vi "temp map test params.vi"() -> ()   [LabVIEW 2009]
uses:
  BME_DG_G05P2/SG05P2 Clock and Trigger Settings.ctl
  LV-BME Interface/BME_DG_TriggerSettings.ctl
  LV-BME Interface/ClockSource.ctl
  LV-BME Interface/BME_DG_V2TriggerSettings.ctl
  ChnlParam.ctl
  Chnl Settings Complete.ctl
  LV-BME Interface/ChnlSettings.ctl
  Go_Done_Chnl_Settings.ctl
  SG08_Chnl_Settings.ctl
  Card Config.ctl
  SG08_Settings.ctl
  POLARIS BME DG.lvlib
panel:
  in  "Advanced Chnl Settings":T1={"Go Signal"=16, "Done Signal"=16} {"Done Signal" format="%04x" items=["Local Primary"=1, "Local Secondary"=2, "Local Force"=4, "Master Primary"=16]; "Go Signal" format="%04x" items=["Local Primary"=1, "Local Secondary"=2, "Local Force"=4, "Resynchronize"=8, "Master Primary"=16, "Master Secondary"=32, "Master Force"=64, "System Clock"=128, "Delay Clock"=256, "Inhibit Local"=512, "Start Local"=1024, "Start Bus"=2048, "Step Back Local"=4096, "Step Back Bus"=8192, "From E"=65536, "From F"=131072, "From Bus"=262144]}
  in  "ChnParameter":T2={" Delay (µs)"=0.0, "On?"=TRUE, "PositiveVoltage?"=TRUE, "50OhmTerminated? "=TRUE, "25OhmOutput?"=FALSE} {"Delay (µs)" min=0.0 max=100000000.0 format="%.5f"}
  out "Card Config":T3[](array[typedef]) {"Advanced Settings"."Trigger on MS Bus" format="%04x" items=["Local Primary"=1, "Local Secondary"=2, "Local Force"=4, "Resynchronize"=8, "Master Primary"=16, "Master Secondary"=32, "Master Force"=64, "System Clock"=128, "Delay Clock"=256, "Inhibit Local"=512, "Start Local"=1024, "Start Bus"=2048, "Step Back Local"=4096, "Step Back Bus"=8192, "Enable From E"=65536, "Enable From F"=131072, "Enable From Bus"=262144]; "Advanced Settings"."Force Trigger (µs)" min=0.0 format="%.6f"; "SG08_Settings"."StepBackTime (µs)" min=0.0 format="%.6f"; "SG08_Settings"."Gate Delay (µs)" format="%.3f"; "SG08_Settings"."Gate Level" min=-2.5 max=2.5 format="%.3g"; "Base Settings"."Gate Divider" min=1 max=1000000; "Base Settings"."Clock Source" items=["Internal Oscillator"=1, "External Trigger"=2, "Trigger-> Oscillator"=3, "MasterSlave Bus"=4]; "Base Settings"."Inhibit(µs)" format="%#_11g"}
  out "Chnl Config":T8[](array[typedef]) {"ChnParameter"."Delay (µs)" min=0.0 max=100000000.0 format="%.5f"; "G08_Chnl_Settings"."Pulse Width (µs)" min=0.0 max=8947840.0 format="%#.6f"; "Go and Done Signal"."Done Signal" format="%04x" items=["Local Primary"=1, "Local Secondary"=2, "Local Force"=4, "Master Primary"=16]; "Go and Done Signal"."Go Signal" format="%04x" items=["Local Primary"=1, "Local Secondary"=2, "Local Force"=4, "Resynchronize"=8, "Master Primary"=16, "Master Secondary"=32, "Master Force"=64, "System Clock"=128, "Delay Clock"=256, "Inhibit Local"=512, "Start Local"=1024, "Start Bus"=2048, "Step Back Local"=4096, "Step Back Bus"=8192, "From E"=65536, "From F"=131072, "From Bus"=262144]}
  in  "ChnlParam":T10[][](array[typedef])=[[{"ChnlName"="Delay Offset", "DelayFormula"=" 10000.0095", "OutputModulo"=1, "Go Signal"=1}, {"ChnlName"="10 Hz Target", "DelayFormula"="Delay Offset - 400", "OutputModulo"=1, "Go Signal"=1}, {"ChnlName"="Fast PC On", "DelayFormula"="Delay Offset", "OutputModulo"=10, "Go Signal"=0}, {"ChnlName"="A2 LDD", "DelayFormula"="Delay Offset-2601", "OutputModulo"=10, "Go Signal"=0}, {"ChnlName"="Oszi", "DelayFormula"="A2 PC On", "OutputModulo"=10, "Go Signal"=0}, {"ChnlName"="A2 PP1 On", "DelayFormula"="A2 PC Off+0.023", "OutputModulo"=10, "Go Signal"=0}, {"ChnlName"="A2 PP2 Off", "DelayFormula"="A2 PP2 On+0.03", "OutputModulo"=10, "Go Signal"=0}, {"ChnlName"="A3 LDD", "DelayFormula"="Delay Offset-2690", "OutputModulo"=100, "Go Signal"=0}, {"ChnlName"="A4 LDD", "DelayFormula"="Delay Offset-2690", "OutputModulo"=400, "Go Signal"=0}], [{"ChnlName"="Pulspicker On", "DelayFormula"="Delay Offset +0.819", "OutputModulo"=10, "Go Signal"=0}, {"ChnlName"="A1 PC On", "DelayFormula"="Pulspicker On+0.009", "OutputModulo"=10, "Go Signal"=0}, {"ChnlName"="Dazzler", "DelayFormula"="A1 PC Off - 36", "OutputModulo"=10, "Go Signal"=0}, {"ChnlName"="A2 PC On", "DelayFormula"="A1 PC Off+0.149", "OutputModulo"=10, "Go Signal"=0}, {"ChnlName"="Kamera", "DelayFormula"="Delay Offset-60", "OutputModulo"=10, "Go Signal"=0}, {"ChnlName"="A2 PP1 Off", "DelayFormula"="A2 PP1 On+0.30", "OutputModulo"=10, "Go Signal"=0}, {"ChnlName"="A2.5 LDD", "DelayFormula"="Delay Offset-2595", "OutputModulo"=50, "Go Signal"=0}, {"ChnlName"="A3 PC On", "DelayFormula"="A2 PC Off+0.172 ", "OutputModulo"=50, "Go Signal"=0}, {"ChnlName"="A3-Kamera", "DelayFormula"="Delay Offset-60", "OutputModulo"=100, "Go Signal"=0}], [{"ChnlName"="Pulspicker Off", "DelayFormula"="Pulspicker On + 0.013", "OutputModulo"=10, "Go Signal"=0}, {"ChnlName"="A1 PC Off", "DelayFormula"="A1 PC On+0.516", "OutputModulo"=10, "Go Signal"=0}, {"ChnlName"="Kompressor", "DelayFormula"="Delay Offset - 100", "OutputModulo"=10, "Go Signal"=0}, {"ChnlName"="A2 PC Off", "DelayFormula"="A2 PC On+0.528", "OutputModulo"=10, "Go Signal"=0}, {"ChnlName"="A5", "DelayFormula"="Delay Offset-2700", "OutputModulo"=800, "Go Signal"=0}, {"ChnlName"="A2 PP2 On", "DelayFormula"="A2 PP1 On+0.003", "OutputModulo"=10, "Go Signal"=0}, {"ChnlName"="Keppis A3", "DelayFormula"="Delay Offset-100", "OutputModulo"=10, "Go Signal"=0}, {"ChnlName"="A3 PC Off", "DelayFormula"="A3 PC On+0.026", "OutputModulo"=50, "Go Signal"=0}, {"ChnlName"="A4-Kamera", "DelayFormula"="Delay Offset-60", "OutputModulo"=400, "Go Signal"=0}]] {"Go Signal" items=["Local Primary"=1, "Local Secondary"=2, "Local Force"=4, "Resynchronize"=8, "Master Primary"=16, "Master Secondary"=32, "Master Force"=64, "System Clock"=128, "Delay Clock"=256, "Inhibit Local"=512, "Start Local"=1024, "Start Bus"=2048, "Step Back Local"=4096, "Step Back Bus"=8192, "From E"=65536, "From F"=131072, "From Bus"=262144]}
  in  "Karten Parameter":T11[](array[typedef])=[{"CardName"="FE PP", "Trigger and Clock"={"Clock Source"=2, " clock devide by"=1, "TriggerEnabled?"=TRUE, "Trigger devide by"=0, "InputTerminated?"=FALSE, "Inhibit(µs)"=99999.9875, "TriggerLevel"=1.4001, "PresetValue"=0, "InternalTrigger?"=TRUE, "InternalArm?"=FALSE, "SWTrigger?"=FALSE, "RisingEdge?"=FALSE, "StopOnPreset?"=FALSE, "ResetWhenDone?"=TRUE, "Gate Divider"=1, "PositiveGate?"=TRUE}, "V2 Trigger Settings"={"Trigger on MS Bus"=1, "Force Trigger (µs)"=0.0, "Gate Type"=TRUE, "Synchronize Gate"=FALSE}}, {"CardName"="A1 Hapt", "Trigger and Clock"={"Clock Source"=4, " clock devide by"=1, "TriggerEnabled?"=TRUE, "Trigger devide by"=0, "InputTerminated?"=FALSE, "Inhibit(µs)"=0.0, "TriggerLevel"=1.0, "PresetValue"=0, "InternalTrigger?"=FALSE, "InternalArm?"=FALSE, "SWTrigger?"=FALSE, "RisingEdge?"=FALSE, "StopOnPreset?"=FALSE, "ResetWhenDone?"=TRUE, "Gate Divider"=1, "PositiveGate?"=TRUE}, "V2 Trigger Settings"={"Trigger on MS Bus"=1, "Force Trigger (µs)"=0.0, "Gate Type"=TRUE, "Synchronize Gate"=FALSE}}, {"CardName"="A1 Neben", "Trigger and Clock"={"Clock Source"=4, " clock devide by"=1, "TriggerEnabled?"=TRUE, "Trigger devide by"=0, "InputTerminated?"=FALSE, "Inhibit(µs)"=0.0, "TriggerLevel"=1.0, "PresetValue"=0, "InternalTrigger?"=FALSE, "InternalArm?"=FALSE, "SWTrigger?"=FALSE, "RisingEdge?"=FALSE, "StopOnPreset?"=FALSE, "ResetWhenDone?"=TRUE, "Gate Divider"=1, "PositiveGate?"=TRUE}, "V2 Trigger Settings"={"Trigger on MS Bus"=1, "Force Trigger (µs)"=0.0, "Gate Type"=TRUE, "Synchronize Gate"=FALSE}}, {"CardName"="A2 Haupt", "Trigger and Clock"={"Clock Source"=4, " clock devide by"=1, "TriggerEnabled?"=TRUE, "Trigger devide by"=0, "InputTerminated?"=FALSE, "Inhibit(µs)"=0.0, "TriggerLevel"=1.0, "PresetValue"=0, "InternalTrigger?"=FALSE, "InternalArm?"=FALSE, "SWTrigger?"=FALSE, "RisingEdge?"=FALSE, "StopOnPreset?"=FALSE, "ResetWhenDone?"=TRUE, "Gate Divider"=1, "PositiveGate?"=TRUE}, "V2 Trigger Settings"={"Trigger on MS Bus"=1, "Force Trigger (µs)"=0.0, "Gate Type"=TRUE, "Synchronize Gate"=FALSE}}, {"CardName"="A2 Neben", "Trigger and Clock"={"Clock Source"=4, " clock devide by"=1, "TriggerEnabled?"=TRUE, "Trigger devide by"=0, "InputTerminated?"=FALSE, "Inhibit(µs)"=0.0, "TriggerLevel"=1.0, "PresetValue"=0, "InternalTrigger?"=FALSE, "InternalArm?"=FALSE, "SWTrigger?"=FALSE, "RisingEdge?"=FALSE, "StopOnPreset?"=FALSE, "ResetWhenDone?"=TRUE, "Gate Divider"=1, "PositiveGate?"=TRUE}, "V2 Trigger Settings"={"Trigger on MS Bus"=1, "Force Trigger (µs)"=0.0, "Gate Type"=TRUE, "Synchronize Gate"=FALSE}}, {"CardName"="A2 PP", "Trigger and Clock"={"Clock Source"=4, " clock devide by"=1, "TriggerEnabled?"=TRUE, "Trigger devide by"=0, "InputTerminated?"=FALSE, "Inhibit(µs)"=0.0, "TriggerLevel"=1.0, "PresetValue"=0, "InternalTrigger?"=FALSE, "InternalArm?"=FALSE, "SWTrigger?"=FALSE, "RisingEdge?"=FALSE, "StopOnPreset?"=FALSE, "ResetWhenDone?"=TRUE, "Gate Divider"=1, "PositiveGate?"=TRUE}, "V2 Trigger Settings"={"Trigger on MS Bus"=1, "Force Trigger (µs)"=0.0, "Gate Type"=TRUE, "Synchronize Gate"=FALSE}}, {"CardName"="A2 PP, A2.5", "Trigger and Clock"={"Clock Source"=4, " clock devide by"=1, "TriggerEnabled?"=TRUE, "Trigger devide by"=0, "InputTerminated?"=FALSE, "Inhibit(µs)"=0.0, "TriggerLevel"=1.0, "PresetValue"=0, "InternalTrigger?"=FALSE, "InternalArm?"=FALSE, "SWTrigger?"=FALSE, "RisingEdge?"=FALSE, "StopOnPreset?"=FALSE, "ResetWhenDone?"=TRUE, "Gate Divider"=1, "PositiveGate?"=TRUE}, "V2 Trigger Settings"={"Trigger on MS Bus"=1, "Force Trigger (µs)"=0.0, "Gate Type"=TRUE, "Synchronize Gate"=FALSE}}, {"CardName"="A3 Haupt", "Trigger and Clock"={"Clock Source"=4, " clock devide by"=1, "TriggerEnabled?"=TRUE, "Trigger devide by"=0, "InputTerminated?"=FALSE, "Inhibit(µs)"=0.0, "TriggerLevel"=1.0, "PresetValue"=0, "InternalTrigger?"=FALSE, "InternalArm?"=FALSE, "SWTrigger?"=FALSE, "RisingEdge?"=FALSE, "StopOnPreset?"=FALSE, "ResetWhenDone?"=TRUE, "Gate Divider"=1, "PositiveGate?"=TRUE}, "V2 Trigger Settings"={"Trigger on MS Bus"=1, "Force Trigger (µs)"=0.0, "Gate Type"=TRUE, "Synchronize Gate"=FALSE}}, {"CardName"="A4 Haupt", "Trigger and Clock"={"Clock Source"=4, " clock devide by"=1, "TriggerEnabled?"=TRUE, "Trigger devide by"=0, "InputTerminated?"=FALSE, "Inhibit(µs)"=0.0, "TriggerLevel"=1.0, "PresetValue"=0, "InternalTrigger?"=FALSE, "InternalArm?"=FALSE, "SWTrigger?"=FALSE, "RisingEdge?"=FALSE, "StopOnPreset?"=FALSE, "ResetWhenDone?"=TRUE, "Gate Divider"=1, "PositiveGate?"=TRUE}, "V2 Trigger Settings"={"Trigger on MS Bus"=1, "Force Trigger (µs)"=0.0, "Gate Type"=TRUE, "Synchronize Gate"=FALSE}}] {"V2 Trigger Settings"."Trigger on MS Bus" format="%04x" items=["Local Primary"=1, "Local Secondary"=2, "Local Force"=4, "Resynchronize"=8, "Master Primary"=16, "Master Secondary"=32, "Master Force"=64, "System Clock"=128, "Delay Clock"=256, "Inhibit Local"=512, "Start Local"=1024, "Start Bus"=2048, "Step Back Local"=4096, "Step Back Bus"=8192, "Enable From E"=65536, "Enable From F"=131072, "Enable From Bus"=262144]; "V2 Trigger Settings"."Force Trigger (µs)" min=0.0 format="%.6f"; "Trigger and Clock"."Gate Divider" min=1 max=1000000; "Trigger and Clock"."Clock Source" items=["Internal Oscillator"=1, "External Trigger"=2, "Trigger-> Oscillator"=3, "MasterSlave Bus"=4]; "Trigger and Clock"."Inhibit(µs)" format="%#_11g"}
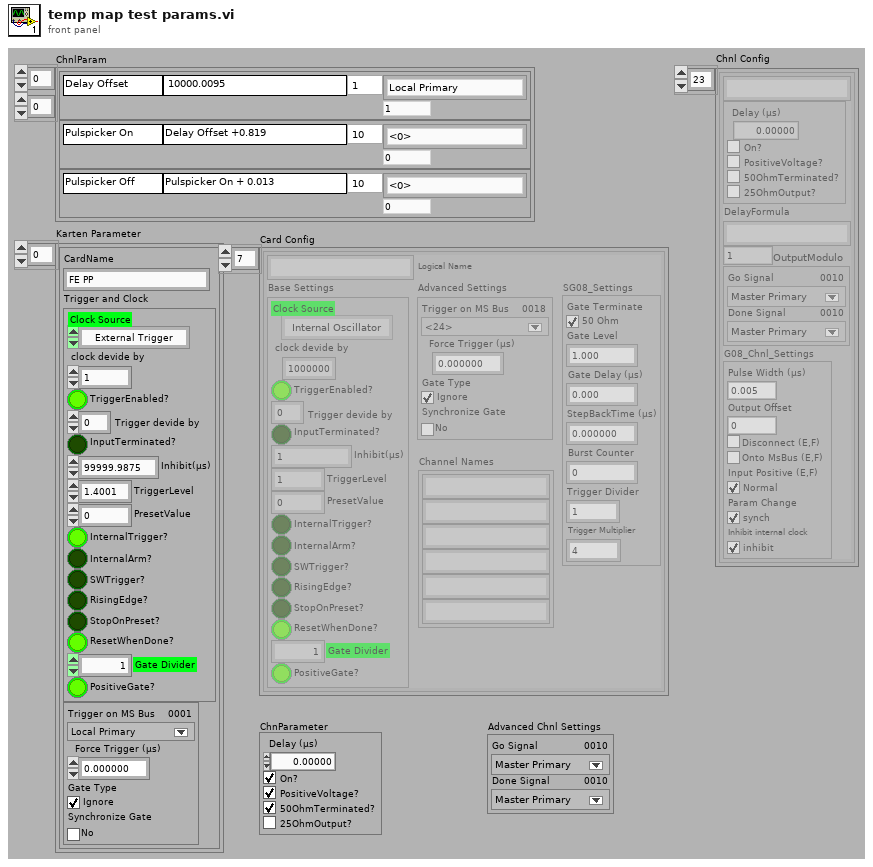
[diagram p1: front panel]
types:
  T1 = typedef "POLARIS BME DG.lvlib/Go_Done_Chnl_Settings.ctl" = cluster{"Go Signal":u32, "Done Signal":u32}
  T2 = typedef "POLARIS BME DG.lvlib/ChnlSettings.ctl" = cluster{" Delay (µs)":dbl, "On?":bool, "PositiveVoltage?":bool, "50OhmTerminated? ":bool, "25OhmOutput?":bool}
  T3 = typedef "POLARIS BME DG.lvlib/Card Config.ctl" = cluster{"Logical Name":string, "Base Settings":T4, "SG08_Settings":T6, "Channel Names":string[], "Advanced Settings":T7}
  T4 = typedef "POLARIS BME DG.lvlib/BME_DG_TriggerSettings.ctl" = cluster{"Clock Source":T5, " clock devide by":u32, "TriggerEnabled?":bool, "Trigger devide by":i32, "InputTerminated?":bool, "Inhibit(µs)":dbl, "TriggerLevel":dbl, "PresetValue":i32, "InternalTrigger?":bool, "InternalArm?":bool, "SWTrigger?":bool, "RisingEdge?":bool, "StopOnPreset?":bool, "ResetWhenDone?":bool, "Gate Divider":i32, "PositiveGate?":bool}
  T5 = typedef "POLARIS BME DG.lvlib/ClockSource.ctl" = i32
  T6 = typedef "POLARIS BME DG.lvlib/SG08_Settings.ctl" = cluster{"Gate Terminate":bool, "Gate Level":dbl, "Gate Delay (µs)":dbl, "StepBackTime (µs)":dbl, "Burst Counter":u32, "Trigger Divider":u32, "Trigger Multiplier":u32}
  T7 = typedef "POLARIS BME DG.lvlib/BME_DG_V2TriggerSettings.ctl" = cluster{"Trigger on MS Bus":u32, "Force Trigger (µs)":dbl, "Gate Type":bool, "Synchronize Gate":bool}
  T8 = typedef "POLARIS BME DG.lvlib/Chnl Settings Complete.ctl" = cluster{"Channel Name":string, "ChnParameter":T2, "DelayFormula":string, "OutputModulo":i32, "Go and Done Signal":T1, "G08_Chnl_Settings":T9}
  T9 = typedef "POLARIS BME DG.lvlib/SG08_Chnl_Settings.ctl" = cluster{"Pulse Width (µs)":dbl, "Output Offset":u32, "Disconnect (E,F)":bool, "Onto MsBus (E,F)":bool, "Input Positive (E,F)":bool, "Param Change":bool, "Inhibit internal clock":bool}
  T10 = typedef "POLARIS BME DG.lvlib/ChnlParam.ctl" = cluster{"ChnlName":string, "DelayFormula":string, "OutputModulo":i32, "Go Signal":u32}
  T11 = typedef "POLARIS BME DG.lvlib/SG05P2 Clock and Trigger Settings.ctl" = cluster{"CardName":string, "Trigger and Clock":T4, "V2 Trigger Settings":T7}
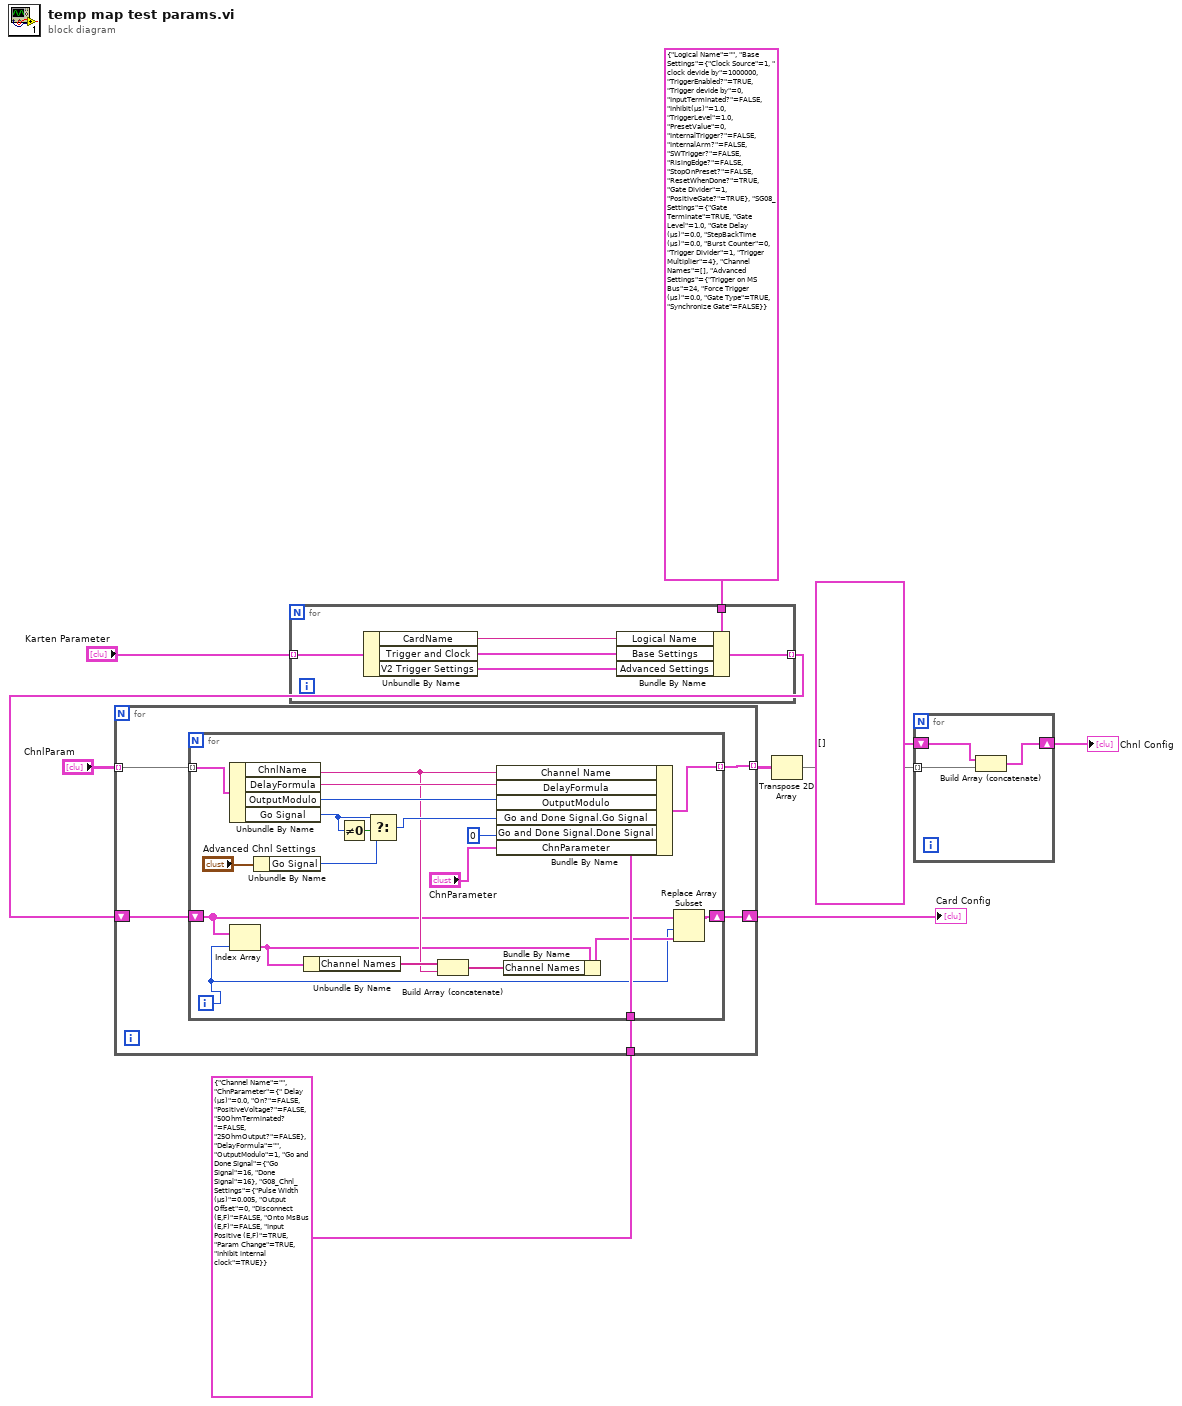
[diagram p0: block diagram]
diagram:
  n1 = for {
    tunnel: "Karten Parameter" -> [w13] mode=indexing
    tunnel: T3 {"Logical Name"="", "Base Settings"={"Clock Source"=1, " clock devide by"=1000000, "TriggerEnabled?"=TRUE, "Trigger devide by"=0, "InputTerminated?"=FALSE, "Inhibit(µs)"=1.0, "TriggerLevel"=1.0, "PresetValue"=0, "InternalTrigger?"=FALSE, "InternalArm?"=FALSE, "SWTrigger?"=FALSE, "RisingEdge?"=FALSE, "StopOnPreset?"=FALSE, "ResetWhenDone?"=TRUE, "Gate Divider"=1, "PositiveGate?"=TRUE}, "SG08_Settings"={"Gate Terminate"=TRUE, "Gate Level"=1.0, "Gate Delay (µs)"=0.0, "StepBackTime (µs)"=0.0, "Burst Counter"=0, "Trigger Divider"=1, "Trigger Multiplier"=4}, "Channel Names"=[], "Advanced Settings"={"Trigger on MS Bus"=24, "Force Trigger (µs)"=0.0, "Gate Type"=TRUE, "Synchronize Gate"=FALSE}} ("Card Config") -> [w12]
    tunnel: [w11] -> w6 mode=indexing
    n2 = Unbundle By Name(w13) -> ("CardName"=w14:string, "Trigger and Clock"=w15:T4, "V2 Trigger Settings"=w16:T7)
    n3 = Bundle By Name(cluster=w12, "Logical Name"=w14, "Base Settings"=w15, "Advanced Settings"=w16) -> (w11:T3)
  }
  n4 = for {
    tunnel: T8 {"Channel Name"="", "ChnParameter"={" Delay (µs)"=0.0, "On?"=FALSE, "PositiveVoltage?"=FALSE, "50OhmTerminated? "=FALSE, "25OhmOutput?"=FALSE}, "DelayFormula"="", "OutputModulo"=1, "Go and Done Signal"={"Go Signal"=16, "Done Signal"=16}, "G08_Chnl_Settings"={"Pulse Width (µs)"=0.005, "Output Offset"=0, "Disconnect (E,F)"=FALSE, "Onto MsBus (E,F)"=FALSE, "Input Positive (E,F)"=TRUE, "Param Change"=TRUE, "Inhibit internal clock"=TRUE}} ("Cluster") -> [w20]
    tunnel: "ChnlParam" -> [w21] mode=indexing
    shift-right: [w18] -> w5
    shift-left: w6 -> [w19]
    tunnel: [w17] -> w4 mode=indexing
    n5 = for {
      tunnel: w21 -> [w41] mode=indexing
      tunnel: [w39] -> w17 mode=indexing
      tunnel: w20 -> [w40]
      shift-right: [w23] -> w18
      shift-left: w19 -> [w25]
      i -> [w22]
      n6 = Unbundle By Name(w41) -> ("ChnlName"=w28:string, "DelayFormula"=w38:string, "OutputModulo"=w37:i32, "Go Signal"=w32:u32)
      n7 = Index Array(array=w25, index=w22) -> (element=w26:T3)
      n8 = Unbundle By Name("Advanced Chnl Settings") -> ("Go Signal"=w30:u32)
      n9 = Unbundle By Name(w26) -> ("Channel Names"=w29:string[])
      n10 = Not Equal To 0?(x=w32) -> (x != 0?=w33:bool)
      n11 = Select(t=w32, s=w33, f=w30) -> (s? t:f=w34:u32)
      n12 = Build Array (concatenate)(w29, w28) -> (w27:string[])
      n13 = Bundle By Name(cluster=w40, "Channel Name"=w28, "DelayFormula"=w38, "OutputModulo"=w37, "Go and Done Signal.Go Signal"=w34, "Go and Done Signal.Done Signal"=u32 0, "ChnParameter"="ChnParameter") -> (w39:T8)
      n14 = Bundle By Name(cluster=w26, "Channel Names"=w27) -> (w24:T3)
      n15 = Replace Array Subset(array=w25, new element=w24, index=w22) -> (w23:T3[])
    }
  }
  "Card Config" <- w5
  n16 = Transpose 2D Array(2D array=w4) -> (transposed array=w3:T8[][])
  n17 = for {
    tunnel: w3 -> [w44] mode=indexing
    shift-right: [w43] -> w2
    shift-left: T8[] [] -> [w42]
    n18 = Build Array (concatenate)(w42, w44) -> (w43:T8[])
  }
  "Chnl Config" <- w2
